vi "SonicShifter.vi"(8 "error in":errorcluster) -> (0 "error out":errorcluster)   [LabVIEW 2015]
uses:
  Sprocket/src/Refname/Queues.ctl
  Sprocket/src/Refname/Actuators.ctl
  Sprocket/src/Action/Action Name.ctl
  Sprocket/src/Refname/Refname to String (Actuator).vi
  Sprocket/src/Refname/Refname to String (Queue).vi
  Sprocket/lib/Sprocket.lvlib
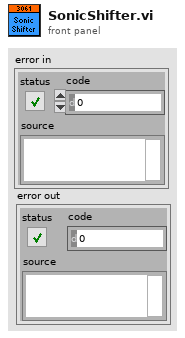
[diagram p1: front panel]
types:
  T1 = typedef "Sprocket.lvlib/Actuators.ctl" = enum16{"Drive Motors L.Top", "Drive Motors R.Top", "Drive Motors L.Bot", "Drive Motors R.Bot", "Collector Motor", "Collector Solenoid", "Compressor", "SonicShifter", "Gyro", "UltraSonic Front Left", "UltraSonic Back Left"}
  T2 = typedef "Sprocket.lvlib/Queues.ctl" = enum16{"Input", "Drive", "Collector", "Shifter"}
  T3 = typedef "WPI_SolenoidDevRef.ctl" = cluster{"DevStatus":errorcluster, "Pneumatics Control Module":u8, "Forward Solenoid Channel":T4, "Reverse Solenoid Channel":T4}
  T4 = typedef "WPI_SolenoidChannel.ctl" = enum8{"Solenoid 0", "Solenoid 1", "Solenoid 2", "Solenoid 3", "Solenoid 4", "Solenoid 5", "Solenoid 6", "Solenoid 7", "Invalid"}
  T5 = typedef "Sprocket.lvlib/Action Name.ctl" = enum16{"No Action", "Drive Train Left", "Drive Train Right", "Drive Train Both", "Collector Motor Eject", "Collector Motor Collect", "Collector Motor Stop", "Collector Extend", "Collector Retract", "Shifter High", "Shifter Low"}
  T6 = typedef "Sprocket.lvlib/Action.ctl" = cluster{"Name":T5, "Priority":i32, "Data":variant}
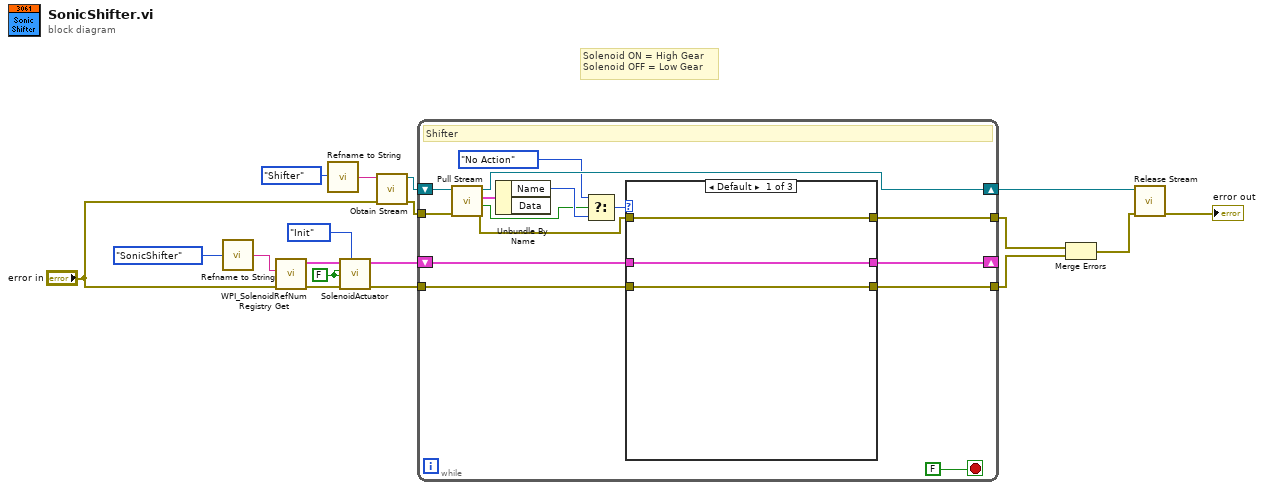
[diagram p0: block diagram]
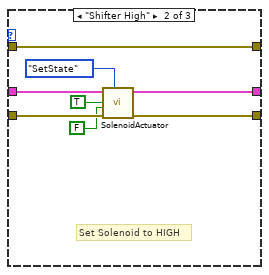
[diagram p2: hidden frame]
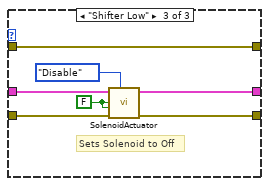
[diagram p3: hidden frame]
diagram:
  w2 = FALSE
  # "Solenoid ON = High Gear\nSolenoid OFF = Low Gear"
  n1 = call-poly "Refname to String.vi"("Actuator Refname"=Actuators."SonicShifter") -> ("Refnum Name"=w9:string)
  n2 = call <vilib>:"WPI_SolenoidRefNum Registry Get.vi"("error in (no error)"="error in", "refnum name"=w9) -> ("error out"=w3:errorcluster, "SolenoidDevRef"=w7:T3)  [unwired: 8 in]
  n3 = call-poly "Refname to String.vi"("Queue Refname"=Queues."Shifter" ("Refname (Queue)")) -> ("Refnum Name"=w11:string)
  n4 = call "SolenoidActuator.vi"("Action"=enum16{"Init", "SetState", "Disable"}."Init", "error in"=w3, "Reverse Actuation"=w2, "Actuate?"=w2, "SolenoidDevRef"=w7) -> ("error out"=w4:errorcluster, "SolenoidDevRef out"=w6:T3)  [unwired: 5 in]
  n5 = call "Obtain Stream.vi"("error in (no error)"="error in", "Name"=w11) -> ("error out"=w15:errorcluster, "stream out"=w14:refnum<queue>)  [unwired: 8 in]
  n6 = while {
    shift-right: [w33] -> w18
    shift-left: w14 -> [w26]
    shift-right: [w19] -> _
    shift-left: w6 -> [w30]
    tunnel: w15 -> [w24]
    tunnel: [w23] -> w1
    tunnel: [w21] -> w17
    tunnel: w4 -> [w20]
    stop <- FALSE stop-if-true
    # "Shifter"
    n7 = call "Pull Stream.vi"("error in (no error)"=w24, "stream in"=w26) -> ("error out"=w22:errorcluster, "timed out?"=w27:bool, "element"=w31:T6, "queue out"=w33:refnum<queue>)  [unwired: 6 in]
    n8 = Unbundle By Name(w31) -> ("Name"=w28:T5)  [unwired: 1 out]
    n9 = Select(t=Action_Name."No Action" ("Name"), s=w27, f=w28) -> (s? t:f=w29:T5)
    n10 = case shown="Default" w29 {
      tunnel: w30 -> [w34 w44 w50]
      tunnel: [w35 w41 w47] -> w23
      tunnel: w22 -> [w36 w37 w45]
      tunnel: [w36 w37 w45] -> w21
      tunnel: w20 -> [w35 w42 w49]
      tunnel: [w34 w43 w48] -> w19
      frame Default {
      }
      frame "Shifter High" {
        # "Set Solenoid to HIGH"
        n11 = call "SolenoidActuator.vi"("Action"=enum16{"Init", "SetState", "Disable"}."SetState", "error in"=w42, "Reverse Actuation"=FALSE, "Actuate?"=TRUE, "SolenoidDevRef"=w44) -> ("error out"=w41:errorcluster, "SolenoidDevRef out"=w43:T3)  [unwired: 5 in]
      }
      frame "Shifter Low" {
        w46 = FALSE
        # "Sets Solenoid to Off"
        n12 = call "SolenoidActuator.vi"("Action"=enum16{"Init", "SetState", "Disable"}."Disable", "error in"=w49, "Reverse Actuation"=w46, "Actuate?"=w46, "SolenoidDevRef"=w50) -> ("error out"=w47:errorcluster, "SolenoidDevRef out"=w48:T3)  [unwired: 5 in]
      }
    }
  }
  n13 = Merge Errors(w17, w1) -> (w16:errorcluster)
  n14 = call "Release Stream.vi"("error in (no error)"=w16, "stream in"=w18) -> ("error out"=→"error out":errorcluster)  [unwired: 8 in, 1 out]
